vi "Caculate 2D Arr Point.vi"(10 "Array":cluster{"X":i32, "Y":i32}, 11 "Set Laser Point Arr":cluster{"Name":string, "X":dbl, "Y":dbl}[][](array[cluster])=[[{"Name"="POINT 1", "X"=0.0, "Y"=0.0}, {"Name"="POINT 2", "X"=0.0, "Y"=0.0}], [{"Name"="POINT 3", "X"=0.0, "Y"=0.0}, {"Name"="POINT 4", "X"=0.0, "Y"=0.0}]]) -> (3 "Laser Point 2D Arr":cluster{"X":sgl, "Y":sgl}[][](array[cluster]))   [LabVIEW 2019]
uses:
  <vilib>/vision/NI_Vision_Development_Module.lvlib
panel:
  out "L24 P":cluster{"X":dbl, "Y":dbl}[](array[cluster])
  out "L34 P":cluster{"X":dbl, "Y":dbl}[](array[cluster])
  out "L13 P":cluster{"X":dbl, "Y":dbl}[](array[cluster])
  out "L12 P":cluster{"X":dbl, "Y":dbl}[](array[cluster])
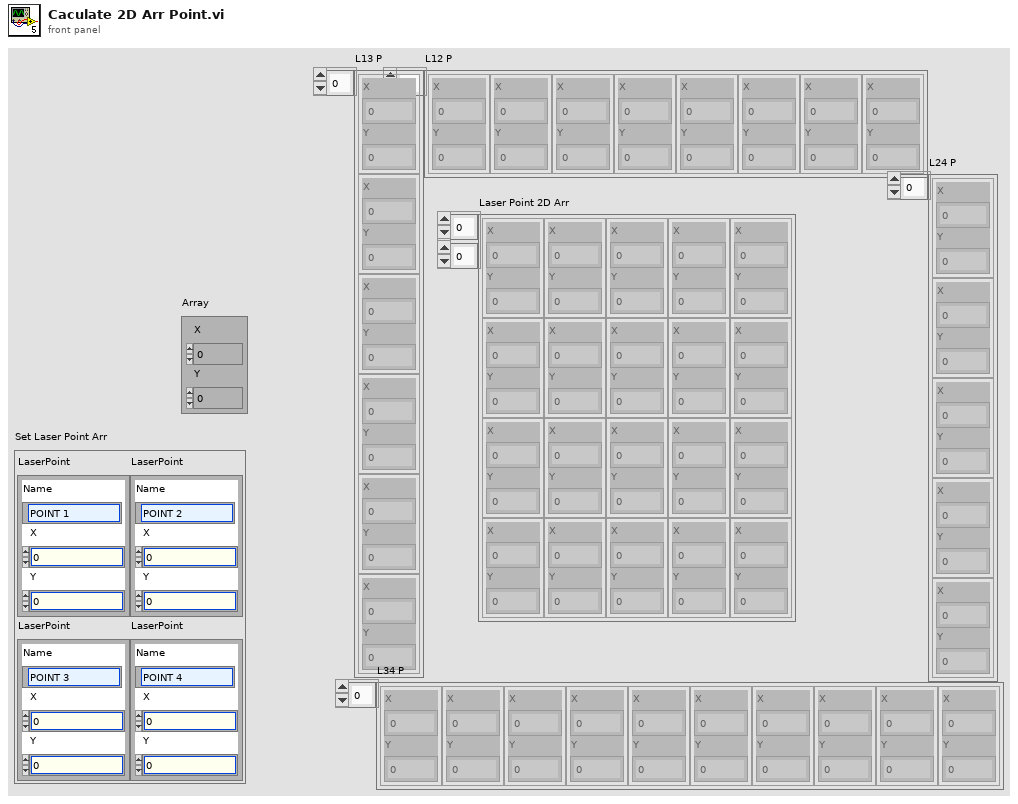
[diagram p1: front panel]
types:
  T1 = cluster{"Point 1":cluster{"X":sgl, "Y":sgl}, "Point 2":cluster{"X":sgl, "Y":sgl}}
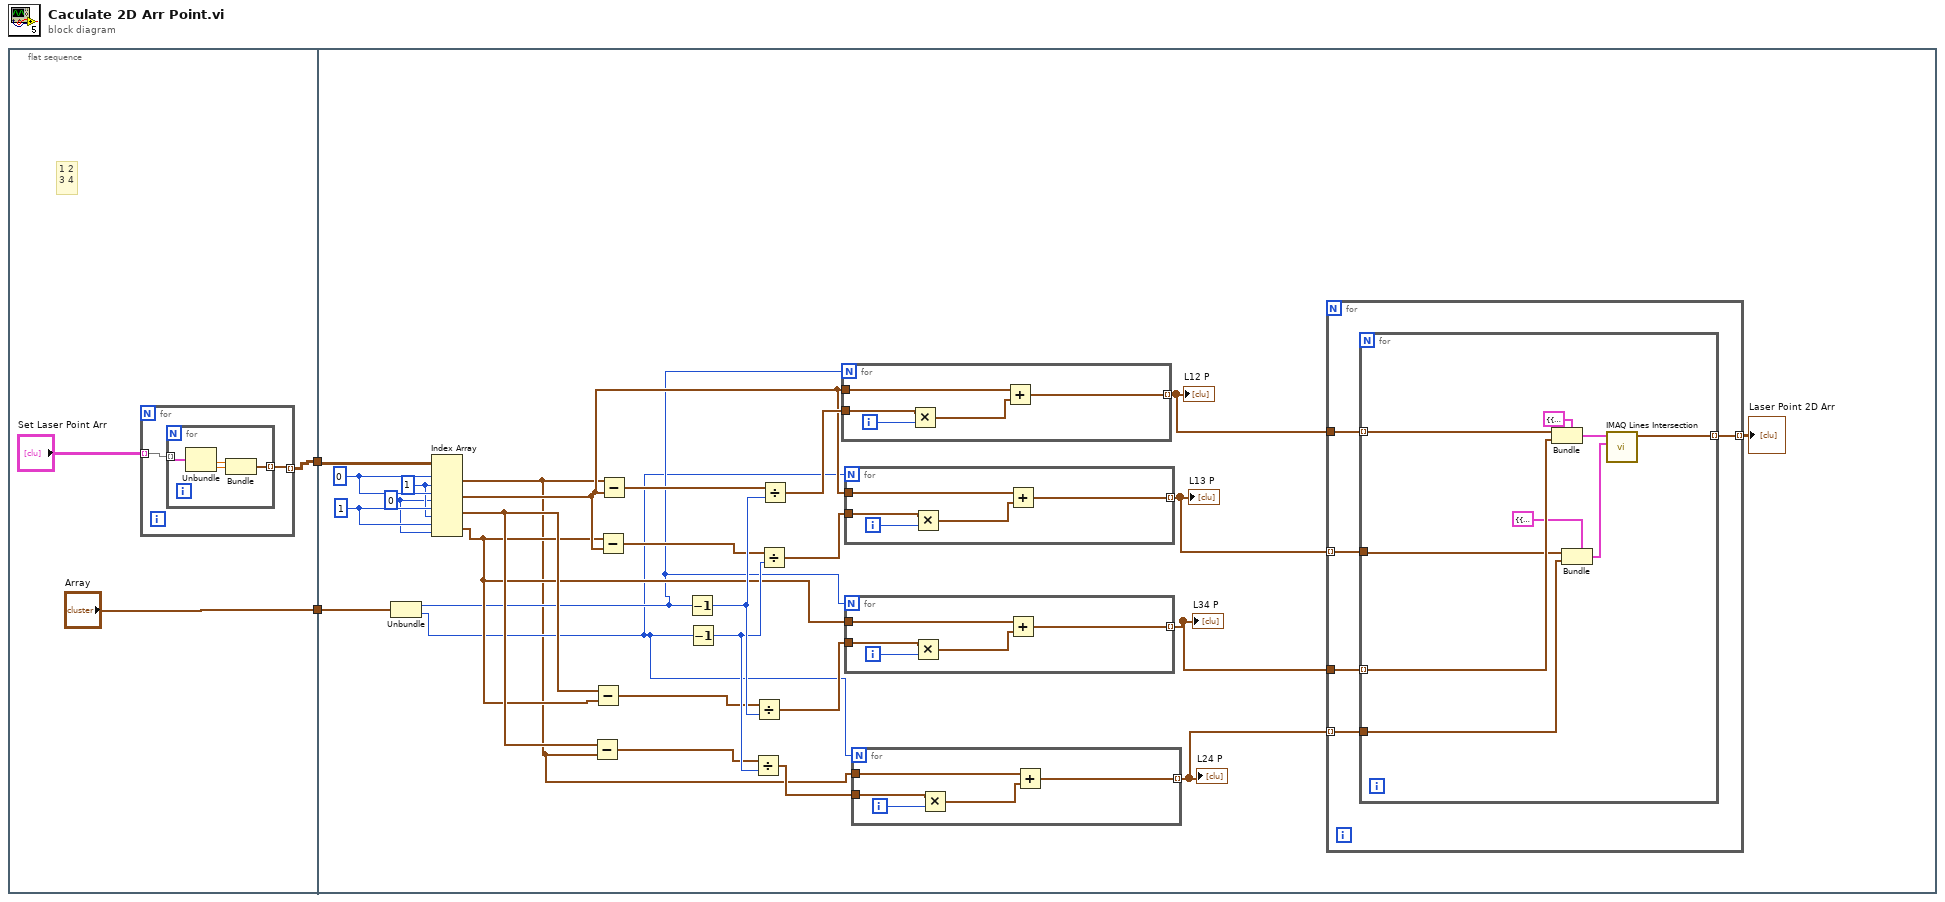
[diagram p0: block diagram]
diagram:
  n1 = flat-sequence {
    tunnel: [w4] -> w2
    tunnel: ["Array"] -> w1
    tunnel: w2 -> [w38]
    tunnel: w1 -> [w33]
    frame #0 {
      # "1 2\n3 4"
      n2 = for {
        tunnel: "Set Laser Point Arr" -> [w7] mode=indexing
        tunnel: [w6] -> w4 mode=indexing
        n3 = for {
          tunnel: w7 -> [w11] mode=indexing
          tunnel: [w8] -> w6 mode=indexing
          n4 = Unbundle(w11) -> ("X"=w10:dbl, "Y"=w9:dbl)  [unwired: 1 out]
          n5 = Bundle("X"=w10, "Y"=w9) -> (w8:cluster{"X":dbl, "Y":dbl})  [unwired: 1 in]
        }
      }
    }
    frame #1 {
      w36 = 1 ("index (row)")
      w34 = 0 ("index (row)")
      w35 = 1 ("index (row)")
      w37 = 0 ("index (row)")
      n6 = Unbundle(w33) -> ("X"=w20:i32, "Y"=w18:i32)
      n7 = Index Array(array=w38, index (row) #1=w37, index (col) #1=w35, index (row) #2=w37, index (col) #2=w34, index (row) #3=w36, index (col) #3=w35, index (row) #4=w36, index (col) #4=w34) -> (element #1=w17:cluster{"X":dbl, "Y":dbl}, element #2=w24:cluster{"X":dbl, "Y":dbl}, element #3=w30:cluster{"X":dbl, "Y":dbl}, element #4=w22:cluster{"X":dbl, "Y":dbl})
      n8 = Subtract(x=w30, y=w17) -> (x-y=w26:cluster{"X":dbl, "Y":dbl})
      n9 = Subtract(x=w30, y=w22) -> (x-y=w27:cluster{"X":dbl, "Y":dbl})
      n10 = Subtract(x=w22, y=w24) -> (x-y=w28:cluster{"X":dbl, "Y":dbl})
      n11 = Subtract(x=w17, y=w24) -> (x-y=w29:cluster{"X":dbl, "Y":dbl})
      n12 = Decrement(x=w20) -> (x-1=w32:i32)
      n13 = Decrement(x=w18) -> (x-1=w31:i32)
      n14 = Divide(x=w26, y=w31) -> (x/y=w19:cluster{"X":dbl, "Y":dbl})
      n15 = Divide(x=w27, y=w32) -> (x/y=w21:cluster{"X":dbl, "Y":dbl})
      n16 = Divide(x=w28, y=w31) -> (x/y=w23:cluster{"X":dbl, "Y":dbl})
      n17 = Divide(x=w29, y=w32) -> (x/y=w25:cluster{"X":dbl, "Y":dbl})
      n18 = for {
        N: w20 -> [_]
        tunnel: w24 -> [w72]
        tunnel: w25 -> [w71]
        tunnel: [w68] -> w16 mode=indexing
        i -> [w70]
        n19 = Multiply(x=w71, y=w70) -> (x*y=w69:cluster{"X":dbl, "Y":dbl})
        n20 = Add(x=w72, y=w69) -> (x+y=w68:cluster{"X":dbl, "Y":dbl})
      }
      "L12 P" <- w16
      n21 = for {
        N: w18 -> [_]
        tunnel: w24 -> [w67]
        tunnel: w23 -> [w66]
        tunnel: [w63] -> w15 mode=indexing
        i -> [w65]
        n22 = Multiply(x=w66, y=w65) -> (x*y=w64:cluster{"X":dbl, "Y":dbl})
        n23 = Add(x=w67, y=w64) -> (x+y=w63:cluster{"X":dbl, "Y":dbl})
      }
      "L13 P" <- w15
      n24 = for {
        N: w20 -> [_]
        tunnel: w22 -> [w62]
        tunnel: w21 -> [w61]
        tunnel: [w58] -> w14 mode=indexing
        i -> [w60]
        n25 = Multiply(x=w61, y=w60) -> (x*y=w59:cluster{"X":dbl, "Y":dbl})
        n26 = Add(x=w62, y=w59) -> (x+y=w58:cluster{"X":dbl, "Y":dbl})
      }
      "L34 P" <- w14
      n27 = for {
        N: w18 -> [_]
        tunnel: w17 -> [w57]
        tunnel: w19 -> [w56]
        tunnel: [w53] -> w13 mode=indexing
        i -> [w55]
        n28 = Multiply(x=w56, y=w55) -> (x*y=w54:cluster{"X":dbl, "Y":dbl})
        n29 = Add(x=w57, y=w54) -> (x+y=w53:cluster{"X":dbl, "Y":dbl})
      }
      "L24 P" <- w13
      n30 = for {
        tunnel: w16 -> [w43]
        tunnel: w15 -> [w42] mode=indexing
        tunnel: w14 -> [w41]
        tunnel: w13 -> [w40] mode=indexing
        tunnel: [w39] -> w12 mode=indexing
        n31 = for {
          tunnel: w43 -> [w51] mode=indexing
          tunnel: w42 -> [w48]
          tunnel: w41 -> [w50] mode=indexing
          tunnel: w40 -> [w47]
          tunnel: [w44] -> w39 mode=indexing
          n32 = Bundle(cluster=T1 {"Point 1"={"X"=0.0, "Y"=0.0}, "Point 2"={"X"=0.0, "Y"=0.0}} ("Line 1"), "Point 1"=w51, "Point 2"=w50) -> (w49:T1)
          n33 = Bundle(cluster=T1 {"Point 1"={"X"=0.0, "Y"=0.0}, "Point 2"={"X"=0.0, "Y"=0.0}} ("Line 2"), "Point 1"=w48, "Point 2"=w47) -> (w46:T1)
          n34 = call "IMAQ Lines Intersection"("Line 2"=w46, "Line 1"=w49) -> ("Intersection Point"=w44:cluster{"X":sgl, "Y":sgl})  [unwired: 7 in, 2 out]
        }
      }
      "Laser Point 2D Arr" <- w12
    }
  }
